vi "Launch App.vi"() -> ()   [LabVIEW 2020]
uses:
  RootActor/RootActor/RootActor.lvclass
  Applications/National Instruments/LabVIEW 2020 64-bit/vi.lib/ActorFramework/Actor/Actor.lvclass
  <vilib>/ActorFramework/Actor/Actor.lvclass
panel:
  out "Progress":u16(slide) scale=0.0..200.0
  # "Actor Application"
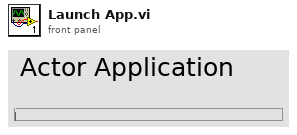
[diagram p1: front panel]
types:
  T1 = enum32{"Invalid", "Standard", "Closed", "Hidden", "Minimized", "Maximized"}
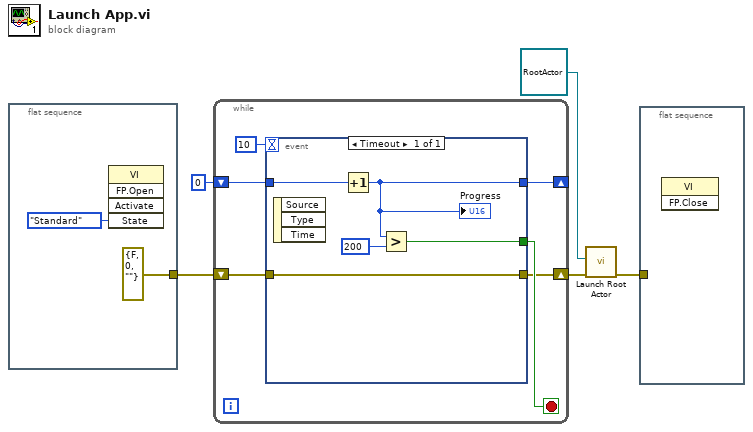
[diagram p0: block diagram]
diagram:
  n1 = flat-sequence {
    tunnel: [errorcluster {"status"=FALSE, "code"=0, "source"=""} ("error constant")] -> w2
    frame #0 {
      n2 = invoke class="VI" method="FP.Open"("State"=T1."Standard") -> ()  [unwired: 4 in, 5 out]
    }
  }
  n3 = while {
    shift-right: [w10] -> _
    shift-left: u16 0 -> [w11]
    shift-right: [w8] -> w3
    shift-left: w2 -> [w13]
    stop <- w9 stop-if-true
    n4 = event shown="[0] Timeout" {
      selector: _ -> [_]
      dyn-events: _ -> [_]
      timeout: 10 -> [_]
      tunnel: w13 -> [w14]
      tunnel: w11 -> [w18]
      tunnel: [w15] -> w10
      tunnel: [w16] -> w9
      tunnel: [w14] -> w8
      event Timeout {
        n5 = event-data() -> ()  [unwired: 1 in, 3 out]
        n6 = Increment(x=w18) -> (x+1=w15:u16)
        "Progress" <- w15
        n7 = Greater?(x=w15, y=u16 200) -> (0:w16:bool)
      }
    }
  }
  n8 = call <vilib>:"Launch Root Actor.vi"("error in (no error)"=w3, "Actor"=refnum<class "RootActor.lvclass"> refnum ("RootActor.lvlib:RootActor.lvclass")) -> ("error out"=w1:errorcluster)  [unwired: 8 in, 1 out]
  n9 = flat-sequence {
    tunnel: w1 -> [_]
    frame #0 {
      n10 = invoke class="VI" method="FP.Close"() -> ()  [unwired: 3 in, 3 out]
    }
  }
